vi "CellColors.vi"() -> (1 "Coerced":u32, 2 "Disabled":u32, 3 "Normal":u32, 5 "True":u32)   [LabVIEW 2018]
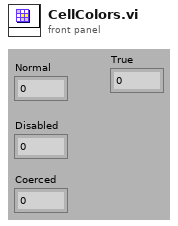
[diagram p1: front panel]
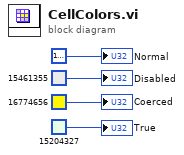
[diagram p0: block diagram]
diagram:
  "Normal" <- u32 16777225
  "Disabled" <- u32 15461355
  "Coerced" <- u32 16774656
  "True" <- u32 15204327
